vi "Rszig számítás.vi"(10 "UIsol":dbl, 11 "U48":dbl) -> (3 "Rszig":dbl)   [LabVIEW 2014]
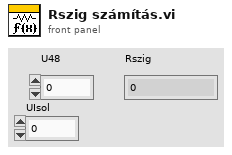
[diagram p1: front panel]
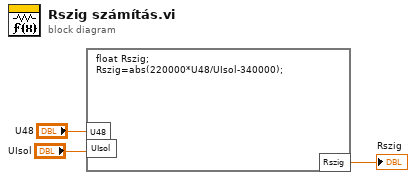
[diagram p0: block diagram]
diagram:
  n1 = formula code="float Rszig;\nRszig=abs(220000*U48/UIsol-340000);"("U48"="U48", "UIsol"="UIsol") -> ("Rszig"=→"Rszig":dbl)
